vi "Data File Processing UI Convert String to Message.vi"(7 "msg in":string) -> (8 "msg":T1)   [LabVIEW 2011]
uses:
  Data File Processing UI Message Define.ctl
  Data File Processing UI Message Type Define.ctl
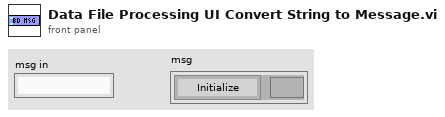
[diagram p1: front panel]
types:
  T1 = typedef "Data File Processing UI Message Define.ctl" = cluster{"data":variant, "type":T2}
  T2 = typedef "Data File Processing UI Message Type Define.ctl" = enum32{"Initialize", "SleepThread", "ErrorHandler", "NoEvent", "PreExit", "Exit", "----Action----", "OpenFile", "SaveFile", "RedrawGraph", "SelectChannel"}
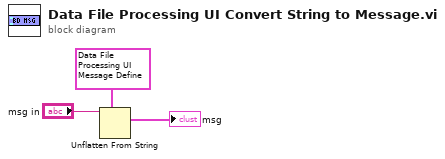
[diagram p0: block diagram]
diagram:
  n1 = Unflatten From String(type=T1 {"data"=variant, "type"=enum."Initialize"} ("MsgDef"), binary string="msg in") -> (value=→"msg":T1)  [unwired: 3 in, 2 out]
